vi "Set Testing.vi"(10 "Testing":bool, 11 "Submission in":refnum<class "Submission.lvclass">) -> (3 "Submission out":refnum<class "Submission.lvclass">)   [LabVIEW 2020, in "Summer of LabVIEW.lvlib" / "Submission.lvclass"]
uses:
  Submission.lvclass
  Submission.lvclass/Submission.ctl
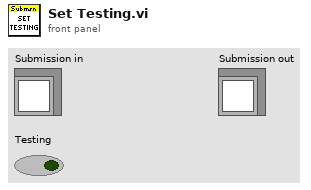
[diagram p1: front panel]
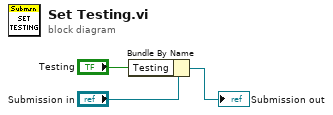
[diagram p0: block diagram]
diagram:
  n1 = Bundle By Name(cluster="Submission in", "Testing"="Testing") -> (→"Submission out":refnum<class "Submission.lvclass">)
